vi "From String.vi"(8 "error in (no error)":errorcluster, 9 "initial scan location":u32, 10 "String":string, 11 "Double Float in":refnum<class "Abs_Time 1D.lvclass">) -> (0 "error out":errorcluster, 1 "offset past scan":u32, 2 "Remaining String":string, 3 "Double Float out":refnum<class "Abs_Time 1D.lvclass">)   [LabVIEW 2021, in "Abs_Time 1D.lvclass"]
uses:
  Abs_Time 1D.lvclass
  C:/TSA/LV_Abstract/Source/Abs_Types/Numeric 1D/Abs_Numeric_1D.lvclass
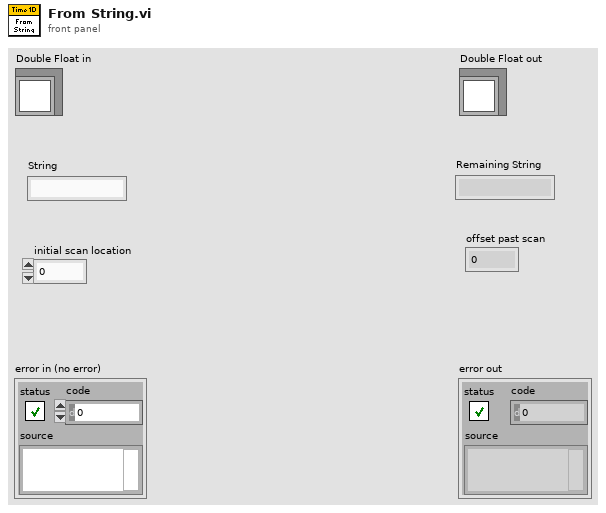
[diagram p1: front panel]
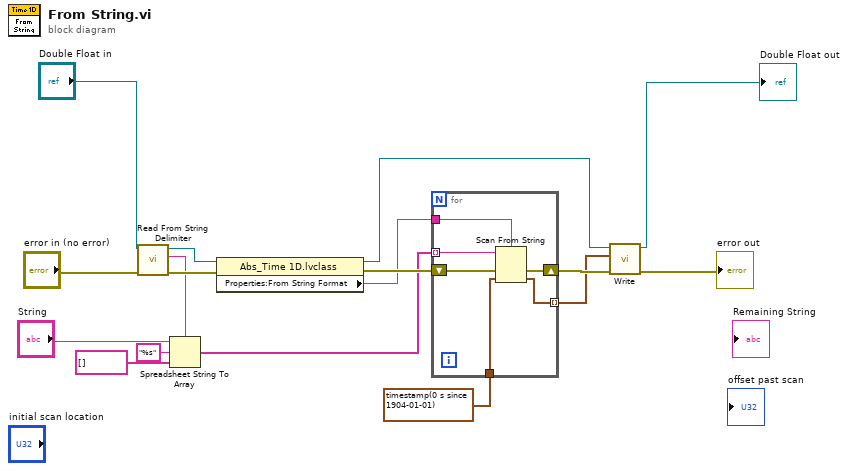
[diagram p0: block diagram]
diagram:
  n1 = call-dynamic "Read From String Delimiter.vi"("error in (no error)"="error in (no error)", "Abs_Array in"="Double Float in") -> ("error out"=w11:errorcluster, "From String Delimiter"=w7:string, "Abs_Array out"=w9:refnum<class "Abs_Time 1D.lvclass">)  [unwired: 7 in]
  n2 = Spreadsheet String To Array(delimiter (Tab)=w7, format string="String", spreadsheet string="%s", array type (2D Dbl)=string[] []) -> (array=w1:string[])
  n3 = property class="Abs_Time 1D.lvclass"(reference=w9, error in=w11) -> (reference out=w13:refnum<class "Abs_Time 1D.lvclass">, error out=w14:errorcluster, "Properties:From String Format"=w2:string)
  n4 = for {
    shift-right: [w23] -> w15
    shift-left: w14 -> [w22]
    tunnel: timestamp(0 s since 1904-01-01) -> [w21]
    tunnel: [w20] -> w3 mode=indexing
    tunnel: w2 -> [w19]
    tunnel: w1 -> [w18] mode=indexing
    n5 = Scan From String(format string=w19, input string=w18, error in=w22, default 1=w21) -> (error out=w23:errorcluster, output 1=w20:timestamp)  [unwired: 1 in, 2 out]
  }
  n6 = call-dynamic "Write.vi"("error in (no error)"=w15, "Value"=w3, "Double Float.lvclass_340760 in"=w13) -> ("error out"=→"error out":errorcluster, "Double Float.lvclass_340760 out"=→"Double Float out":refnum<class "Abs_Time 1D.lvclass">)  [unwired: 7 in]
